vi "States 2 Leds.vi"(10 "MixedModeStates":T1) -> (2 "Mixed Mode State Display":T2)   [LabVIEW 2009]
uses:
  Mixed Mode State Display.ctl
  Mixed Mode States.ctl
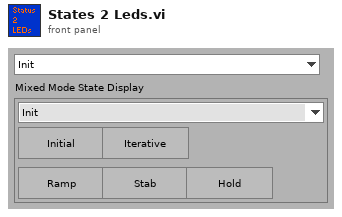
[diagram p1: front panel]
types:
  T1 = typedef "Mixed Mode States.ctl" = enum16{"Init", "Idle", "Start Initial Ramp", "Run Initial Ramp", "Start Iterative Stage", "Convergence Check", "Update Stiffness Jacobian", "Update Command", "Start Iterative Ramp", "Run Iterative Ramp", "Start Iterative Stabilize", "Iterative Stabilize", "Start Iterative Holding", "Iterative Holding", "Start Stabilize", "Stabilize", "Start Hold", "Holding", "Done", "Aborting", "Exit", "Nop"}
  T2 = typedef "Mixed Mode State Display.ctl" = cluster{"MixedModeStates":T1, "Initial":bool, "Iterative":bool, "Ramp":bool, "Stab":bool, "Hold":bool}
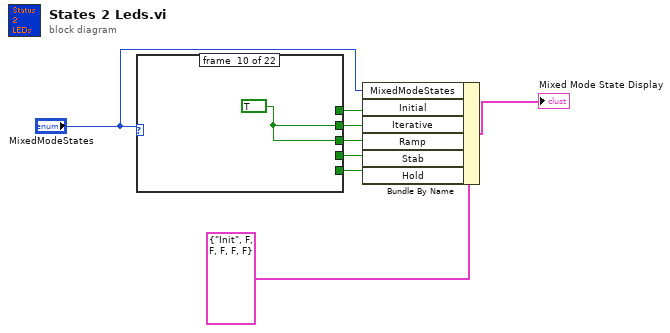
[diagram p0: block diagram]
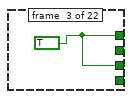
[diagram p4: hidden frame]
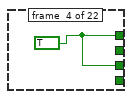
[diagram p5: hidden frame]
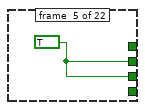
[diagram p6: hidden frame]
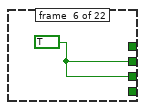
[diagram p7: hidden frame]
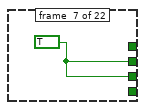
[diagram p8: hidden frame]
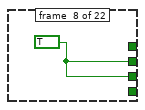
[diagram p9: hidden frame]
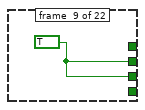
[diagram p10: hidden frame]
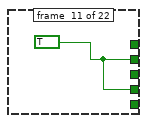
[diagram p11: hidden frame]
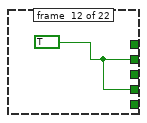
[diagram p12: hidden frame]
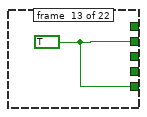
[diagram p13: hidden frame]
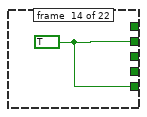
[diagram p14: hidden frame]
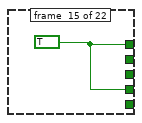
[diagram p15: hidden frame]
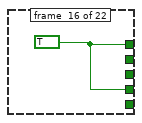
[diagram p16: hidden frame]
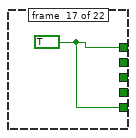
[diagram p17: hidden frame]
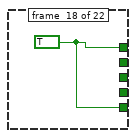
[diagram p18: hidden frame]
diagram:
  n1 = case shown="\"Nop\"" "MixedModeStates" {
    tunnel: [_ _ w9 w10 _ _ _ _ _ _ _ _ _ _ w21 w22 w23 w24 _ _ _ _] -> w5
    tunnel: [_ _ w9 w10 w11 w12 w13 w14 w15 w16 _ _ _ _ _ _ _ _ _ _ _ _] -> w4
    tunnel: [_ _ _ _ w11 w12 w13 w14 w15 w16 w17 w18 w19 w20 _ _ _ _ _ _ _ _] -> w3
    tunnel: [_ _ _ _ _ _ _ _ _ _ w17 w18 _ _ w21 w22 _ _ _ _ _ _] -> w2
    tunnel: [_ _ _ _ _ _ _ _ _ _ _ _ w19 w20 _ _ w23 w24 _ _ _ _] -> w1
    frame #0 {
    }
    frame #1 {
    }
    frame #2 {
      w9 = TRUE
    }
    frame #3 {
      w10 = TRUE
    }
    frame #4 {
      w11 = TRUE
    }
    frame #5 {
      w12 = TRUE
    }
    frame #6 {
      w13 = TRUE
    }
    frame #7 {
      w14 = TRUE
    }
    frame #8 {
      w15 = TRUE
    }
    frame #9 {
      w16 = TRUE
    }
    frame #10 {
      w17 = TRUE
    }
    frame #11 {
      w18 = TRUE
    }
    frame #12 {
      w19 = TRUE
    }
    frame #13 {
      w20 = TRUE
    }
    frame #14 {
      w21 = TRUE
    }
    frame #15 {
      w22 = TRUE
    }
    frame #16 {
      w23 = TRUE
    }
    frame #17 {
      w24 = TRUE
    }
    frame #18 {
    }
    frame #19 {
    }
    frame #20 {
    }
    frame #21 {
    }
  }
  n2 = Bundle By Name(cluster=T2 {"MixedModeStates"=enum."Init", "Initial"=FALSE, "Iterative"=FALSE, "Ramp"=FALSE, "Stab"=FALSE, "Hold"=FALSE} ("Mixed Mode State Display"), "MixedModeStates"="MixedModeStates", "Initial"=w5, "Iterative"=w3, "Ramp"=w4, "Stab"=w2, "Hold"=w1) -> (→"Mixed Mode State Display":T2)
